vi "INIboolean.vi"(7 "Section":string, 8 "error in (no error)":errorcluster, 9 "default value":bool, 10 "Key":string, 11 "Refnum in":T1) -> (0 "Error Out":errorcluster, 1 "Value":bool, 3 "Refnum out":T1)   [LabVIEW 2013]
uses:
  <vilib>/Utility/config.llb/Config Data RefNum.ctl
  <vilib>/Utility/config.llb/Read Key (Boolean).vi
  <vilib>/Utility/config.llb/Write Key (Boolean).vi
  <vilib>/Utility/config.llb/NI_LVConfig.lvlib
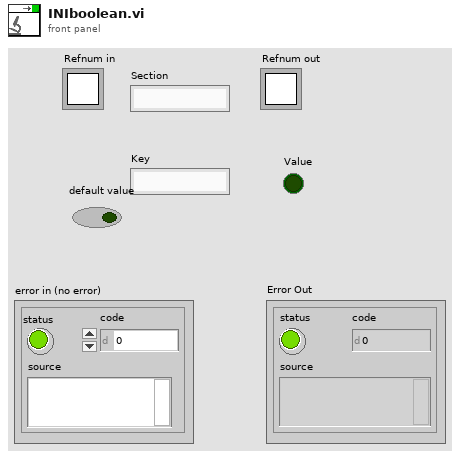
[diagram p1: front panel]
types:
  T1 = typedef "NI_LVConfig.lvlib/Config Data RefNum.ctl" = refnum<k1>
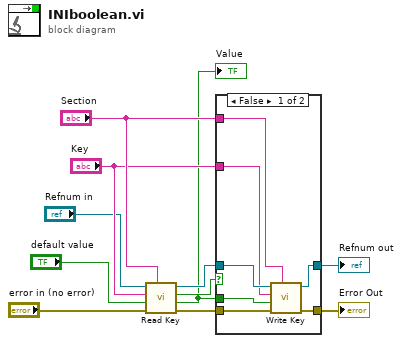
[diagram p0: block diagram]
diagram:
  n1 = call-poly <vilib>:"Read Key.vi"("section"="Section", "error in (no error)"="error in (no error)", "default value"="default value", "key"="Key", "refnum"="Refnum in") -> ("error out"=w6:errorcluster, "value"=w1:bool, "found?"=w4:bool, "refnum out"=w5:T1)  [unwired: 3 in]
  "Value" <- w1
  n2 = case shown="False" w4 {
    tunnel: [w17 w20] -> w10
    tunnel: w5 -> [w18 w20]
    tunnel: w1 -> [w16 _]
    tunnel: w6 -> [w15 w19]
    tunnel: [w14 w19] -> w3
    tunnel: "Section" -> [w13 _]
    tunnel: "Key" -> [w12 _]
    frame False {
      n3 = call-poly <vilib>:"Write Key.vi"("section"=w13, "error in (no error)"=w15, "value"=w16, "key"=w12, "refnum"=w18) -> ("error out"=w14:errorcluster, "refnum out"=w17:T1)  [unwired: 4 in, 1 out]
    }
    frame True {
    }
  }
  "Refnum out" <- w10
  "Error Out" <- w3
